vi "BoxVariant.vi"(10 "Variant":variant) -> (2 "Variant Out":refnum<class "Variant.lvclass">)   [LabVIEW 2013, in "LapDog.Collections.v_.Common.lvlib" / "Variant.lvclass"]
uses:
  Variant.lvclass
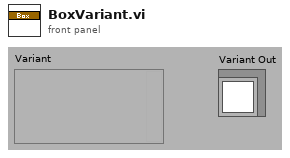
[diagram p1: front panel]
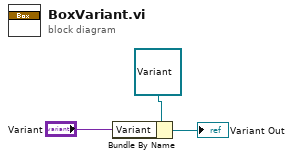
[diagram p0: block diagram]
diagram:
  n1 = Bundle By Name(cluster=refnum<class "Variant.lvclass"> refnum ("LapDog.Collections.v0.Lists.Interfaces.lvlib:String.lvclass"), "Variant"="Variant") -> (→"Variant Out":refnum<class "Variant.lvclass">)
